vi "TimingVIHelp.vi"(4 "Help File Name":string="lvfpga.chm", 5 "String":string) -> (0 "error out":errorcluster)   [LabVIEW 2017]
doc: "This is a placeholder VI that later will be used to link to the on-line help for the timing VIs"
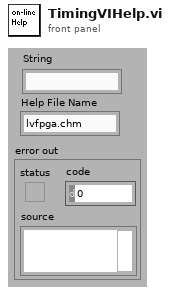
[diagram p1: front panel]
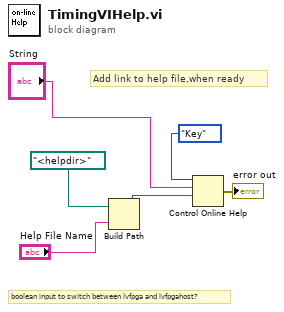
[diagram p0: block diagram]
diagram:
  # "boolean input to switch between lvfpga and lvfpgahost?"
  # "Add link to help file,when ready"
  n1 = Build Path(base path=path "<helpdir>" ("Application:Directory Path"), name or relative path="Help File Name") -> (appended path=w3:path)
  n2 = Control Online Help(2:w3, 3:"String", 4:enum16{"Contents", "Key", "Close"}."Key" ("Operation")) -> (0:→"error out":errorcluster)  [unwired: 1 in]
